vi "lifetimeExport.vi"(4 "Cursor List":T1, 5 "histogram 3":dbl[](array[numeric]), 6 "histogram 2":dbl[](array[numeric]), 7 "histogram 1":dbl[](array[numeric]), 8 "time in":dbl[](array[numeric])) -> (0 "histogram 3 out":dbl[](array[numeric]), 1 "histogram2 out":dbl[](array[numeric]), 2 "histogram 1 out":dbl[](array[numeric]), 3 "time out":dbl[](array[numeric]))   [LabVIEW 2009]
uses:
  <vilib>/Utility/miscctls.llb/LVCursorListTypeDef.ctl
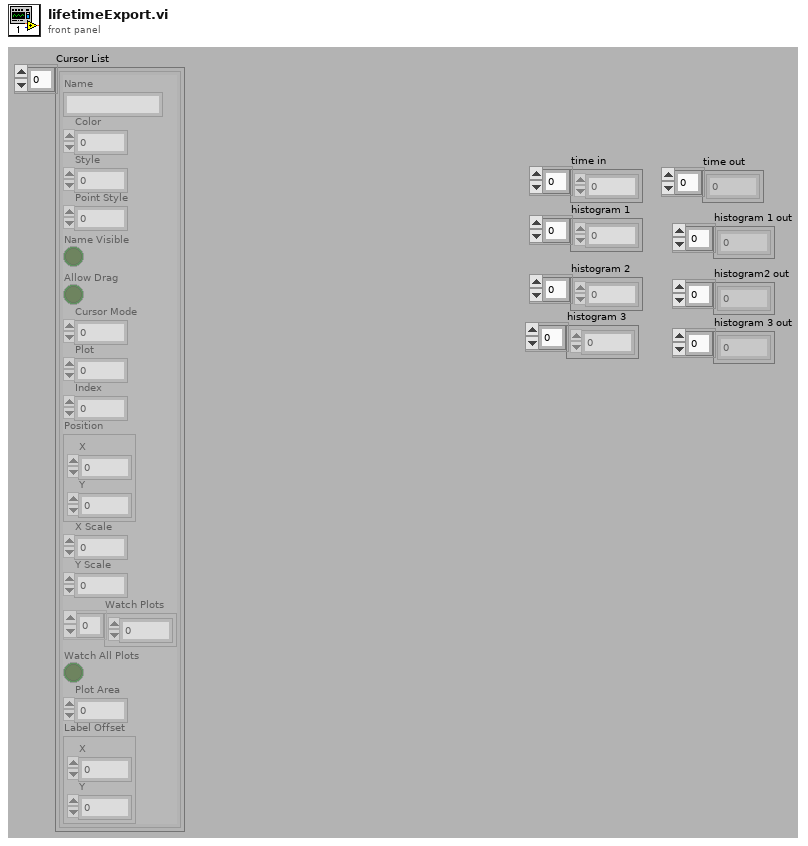
[diagram p1: front panel]
types:
  T1 = typedef "LVCursorListTypeDef.ctl" = cluster{"Name":string, "Color":u32, "Style":u8, "Point Style":u8, "Name Visible":bool, "Allow Drag":bool, "Cursor Mode":u32, "Plot":i32, "Index":i32, "Position":cluster{"X":dbl, "Y":dbl}, "X Scale":u32, "Y Scale":u32, "Watch Plots":i32[], "Watch All Plots":bool, "Plot Area":i32, "Label Offset":cluster{"X":dbl, "Y":dbl}}[]
  T2 = cluster{"Name":string, "Color":u32, "Style":u8, "Point Style":u8, "Name Visible":bool, "Allow Drag":bool, "Cursor Mode":u32, "Plot":i32, "Index":i32, "Position":cluster{"X":dbl, "Y":dbl}, "X Scale":u32, "Y Scale":u32, "Watch Plots":i32[], "Watch All Plots":bool, "Plot Area":i32, "Label Offset":cluster{"X":dbl, "Y":dbl}}
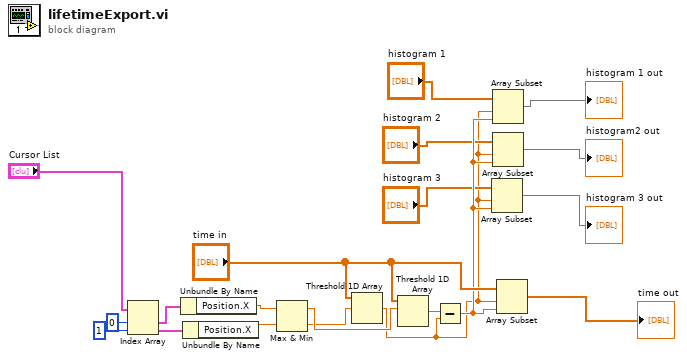
[diagram p0: block diagram]
diagram:
  n1 = Index Array(array="Cursor List", index #1=0 ("Index"), index #2=1 ("Index")) -> (element #1=w14:T2, element #2=w15:T2)
  n2 = Unbundle By Name(w14) -> ("Position.X"=w16:dbl)
  n3 = Unbundle By Name(w15) -> ("Position.X"=w17:dbl)
  n4 = Max & Min(x=w16, y=w17) -> (max(x,y)=w19:dbl, min(x,y)=w18:dbl)
  n5 = Threshold 1D Array(2:w18, 3:"time in") -> (0:w3:dbl)  [unwired: 1 in]
  n6 = Threshold 1D Array(2:w19, 3:"time in") -> (0:w4:dbl)  [unwired: 1 in]
  n7 = Subtract(x=w4, y=w3) -> (x-y=w11:dbl)
  n8 = Array Subset(array="histogram 3", index=w3, length=w11) -> (→"histogram 3 out":dbl[])
  n9 = Array Subset(array="histogram 1", index=w3, length=w11) -> (→"histogram 1 out":dbl[])
  n10 = Array Subset(array="histogram 2", index=w3, length=w11) -> (→"histogram2 out":dbl[])
  n11 = Array Subset(array="time in", index=w3, length=w11) -> (→"time out":dbl[])
